vi "Test Namer with Folder creates folder.vi"   [LabVIEW 2020, in "Namer.Tests.lvclass"]
uses:
  Namer.Tests.lvclass
  Source/Approval Tests/Namer with Folder/Namer with Folder.lvclass
  Source/Approval Tests/Naming Data/Naming Data.lvclass
  Source/Approval Tests/Naming Data/Naming Data.lvclass/Naming Data.ctl
  Source/Approval Tests/Naming Data/Write Test VI Name.vi
  <vilib>/addons/_JKI Toolkits/Caraya/classes/Assert/Assert False.vi
  <vilib>/addons/_JKI Toolkits/Caraya/classes/Assert/Assert True.vi
  <vilib>/addons/_JKI Toolkits/Caraya/classes/Test/Test.lvclass
  <vilib>/addons/_JKI Toolkits/Caraya/classes/Assert/Assert.lvclass
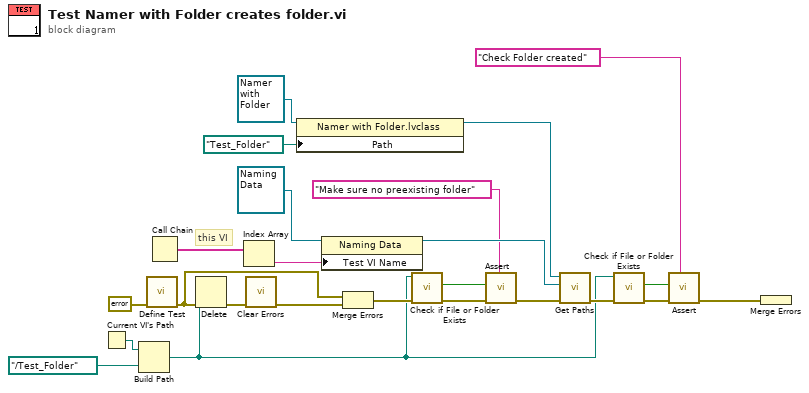
[diagram p0: block diagram]
diagram:
  # "this VI"
  n1 = Current VI's Path() -> (path=w13:path)
  n2 = Build Path(base path=w13, name or relative path=path "../Test_Folder") -> (appended path=w3:path)
  n3 = call <vilib>:"Define Test.vi"("error in (no error)"=errorcluster {"status"=FALSE, "code"=0, "source"=""}) -> ("error out"=w12:errorcluster)  [unwired: 9 in, 1 out]
  n4 = Call Chain() -> (call chain=w21:string[])
  n5 = Delete(path (use dialog)=w3, error in=w12) -> (error out=w11:errorcluster)  [unwired: 3 in, 2 out]
  n6 = Index Array(array=w21) -> (element=w20:string)  [unwired: 1 in]
  n7 = call <vilib>:"Clear Errors.vi"("error in (no error)"=w11) -> ("error out"=w10:errorcluster)  [unwired: 5 in, 1 out]
  n8 = property class="Namer with Folder.lvclass"(reference=refnum<class "Namer with Folder.lvclass"> refnum ("Approval Tests:Namer with Folder.lvclass"), "Path"=path "Test_Folder") -> (reference out=w16:refnum<class "Namer with Folder.lvclass">)  [unwired: 1 in, 1 out]
  n9 = property on="Property Node" class="Naming Data"(reference=refnum<class "Naming Data.lvclass"> refnum ("Naming Data"), "Test VI Name"=w20) -> (reference out=w19:refnum<class "Naming Data.lvclass">)  [unwired: 1 in, 1 out]
  n10 = Merge Errors(w12, w10) -> (w8:errorcluster)
  n11 = call <vilib>:"Check if File or Folder Exists.vi"("error in (no error)"=w8, "path"=w3) -> ("error out"=w4:errorcluster, "file or folder exists?"=w2:bool)  [unwired: 7 in, 1 out]
  n12 = call-poly <vilib>:"Assert.vi"("Label"="Make sure no preexisting folder", "error in (no error)"=w4, "False?"=w2) -> ("error out"=w5:errorcluster)  [unwired: 7 in, 1 out]
  n13 = call-dynamic "Get Paths.vi"("error in"=w5, "Naming Data"=w19, "Namer with Folder in"=w16) -> ("error out"=w9:errorcluster)  [unwired: 5 in, 3 out]
  n14 = call <vilib>:"Check if File or Folder Exists.vi"("error in (no error)"=w9, "path"=w3) -> ("error out"=w7:errorcluster, "file or folder exists?"=w6:bool)  [unwired: 7 in, 1 out]
  n15 = call-poly <vilib>:"Assert.vi"("Label"="Check Folder created" ("Label (VI Title)"), "error in (no error)"=w7, "True?"=w6) -> ("error out"=w18:errorcluster)  [unwired: 7 in, 1 out]
  n16 = Merge Errors(w18) -> ()  [unwired: 1 out]
